vi "SCCSup RemoveDupPathsInArray.vi"(2 "sort? (T)":bool=TRUE, 7 "path array in":path[](array[path])) -> (8 "path array out":path[](array[path]))   [LabVIEW 2017]
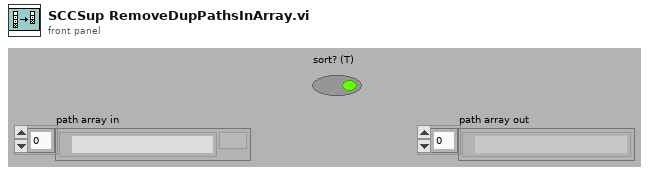
[diagram p1: front panel]
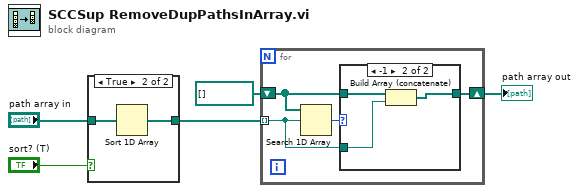
[diagram p0: block diagram]
diagram:
  n1 = case shown="True" "sort? (T)" {
    tunnel: "path array in" -> [w6 w8]
    tunnel: [w6 w7] -> w4
    frame False {
    }
    frame True {
      n2 = Sort 1D Array(array=w8) -> (sorted array=w7:path[])
    }
  }
  n3 = for {
    tunnel: w4 -> [w9] mode=indexing
    shift-right: [w10] -> w3
    shift-left: path[] [] -> [w11]
    n4 = Search 1D Array(1D array=w11, element=w9) -> (index of element=w12:i32)  [unwired: 1 in]
    n5 = case shown="-1" w12 {
      tunnel: w11 -> [w13 w16]
      tunnel: [w13 w15] -> w10
      tunnel: w9 -> [_ w14]
      frame Default {
      }
      frame -1 {
        n6 = Build Array (concatenate)(w16, w14) -> (w15:path[])
      }
    }
  }
  "path array out" <- w3
